vi "Drive PID.vi"(11 "Process Variable":dbl format="%.2f") -> (3 "Output":dbl format="%.2f")   [LabVIEW 2013]
uses:
  <vilib>/Rock Robotics/WPI/DriverStation/WPI_DriverStationRobotMode2.ctl
  Begin/Robot Global Data.vi
  <vilib>/addons/control/pid/pid.llb/PID (DBL).vi
  <vilib>/addons/control/pid/NI_PID_pid.lvlib
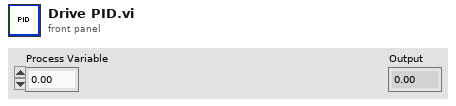
[diagram p1: front panel]
types:
  T1 = typedef "WPI_DriverStationRobotMode2.ctl" = enum16{"Autonomous Disabled", "Autonomous Enabled", "Teleop Disabled", "Teleop Enabled", "Timeout", "Finish", "Test Disabled", "Test Enabled"}
  T2 = cluster{"proportional gain (Kc)":dbl, "integral time (Ti, min)":dbl, "derivative time (Td, min)":dbl}
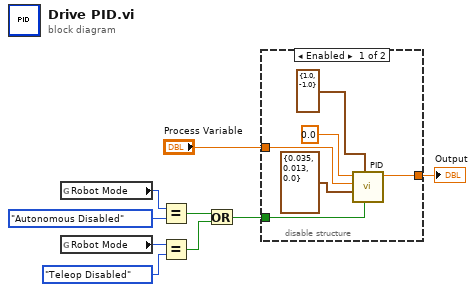
[diagram p0: block diagram]
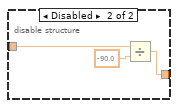
[diagram p2: hidden frame]
diagram:
  n1 = global read "Robot Global Data.vi" "Robot Mode"() -> (w7:T1)
  n2 = global read "Robot Global Data.vi" "Robot Mode"() -> (w4:T1)
  n3 = Equal?(x=w7, y=WPI_DriverStationRobotMode2."Autonomous Disabled" ("Robot Mode")) -> (x = y?=w3:bool)
  n4 = Equal?(x=w4, y=WPI_DriverStationRobotMode2."Teleop Disabled" ("Robot Mode")) -> (x = y?=w2:bool)
  n5 = Or(x=w3, y=w2) -> (x .or. y?=w1:bool)
  n6 = disable-structure shown="Enabled" {
    disable-tunnel: "Process Variable" -> [w13 w18]
    disable-tunnel: [w11 w16] -> w8
    disable-tunnel: w1 -> [w10 _]
    frame Enabled {
      n7 = call-poly <vilib>:"PID.vi"("reinitialize? (F)"=w10, "output range"=cluster{"output high":dbl, "output low":dbl} {"output high"=1.0, "output low"=-1.0}, "PID gains"=T2 {"proportional gain (Kc)"=0.035, "integral time (Ti, min)"=0.013, "derivative time (Td, min)"=0.0}, "process variable"=w13, "setpoint"=0.0) -> ("output"=w11:dbl)  [unwired: 5 in, 1 out]
    }
    frame Disabled {
      n8 = Divide(x=w18, y=-90.0) -> (x/y=w16:dbl)
    }
  }
  "Output" <- w8
